vi "colorBool.vi"(6 "GObj Refnum":refnum<vi>, 9 "GObj Refnum 2":refnum<vi>, 10 "GObj Refnum 3":refnum<vi>, 11 "GObject in":refnum<vi>) -> (3 "Boolean":bool)   [LabVIEW 2014]
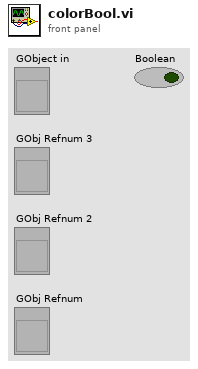
[diagram p1: front panel]
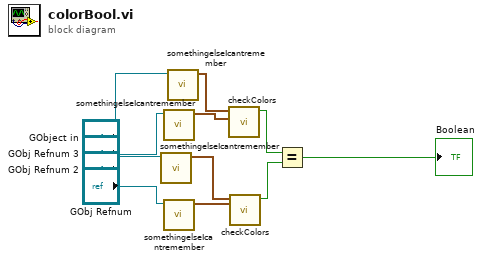
[diagram p0: block diagram]
diagram:
  n1 = call "somethingelseIcantremember.vi"("GObject in"="GObj Refnum 2") -> ("Colors [4]"=w7:cluster{u32, u32}[])  [unwired: 10 in]
  n2 = call "somethingelseIcantremember.vi"("GObject in"="GObj Refnum 3") -> ("Colors [4]"=w6:cluster{u32, u32}[])  [unwired: 10 in]
  n3 = call "somethingelseIcantremember.vi"("GObject in"="GObj Refnum") -> ("Colors [4]"=w8:cluster{u32, u32}[])  [unwired: 10 in]
  n4 = call "somethingelseIcantremember.vi"("GObject in"="GObject in") -> ("Colors [4]"=w5:cluster{u32, u32}[])  [unwired: 10 in]
  n5 = call "checkColors.vi"("Colors [4]"=w6, "Array"=w5) -> ("Boolean"=w9:bool)  [unwired: 9 in]
  n6 = call "checkColors.vi"("Colors [4]"=w8, "Array"=w7) -> ("Boolean"=w10:bool)  [unwired: 9 in]
  n7 = Equal?(x=w9, y=w10) -> (x = y?=→"Boolean":bool)
